vi "HeaderBis.vi"(0 "UUTHeader":string, 1 "ProductRev":string, 2 "P/N UUT":string, 3 "DSP SN":string, 5 "Driver S/N":string, 6 "error in":errorcluster, 10 "UA":string, 11 "VR":string, 12 "POWER SN":string, 13 "Oper.":string, 16 "Revision Param":string, 17 "Tester Software Ver":string) -> (20 "table header":string, 22 "Array":string[][](array[string]), 26 "error out":errorcluster)   [LabVIEW 2017]
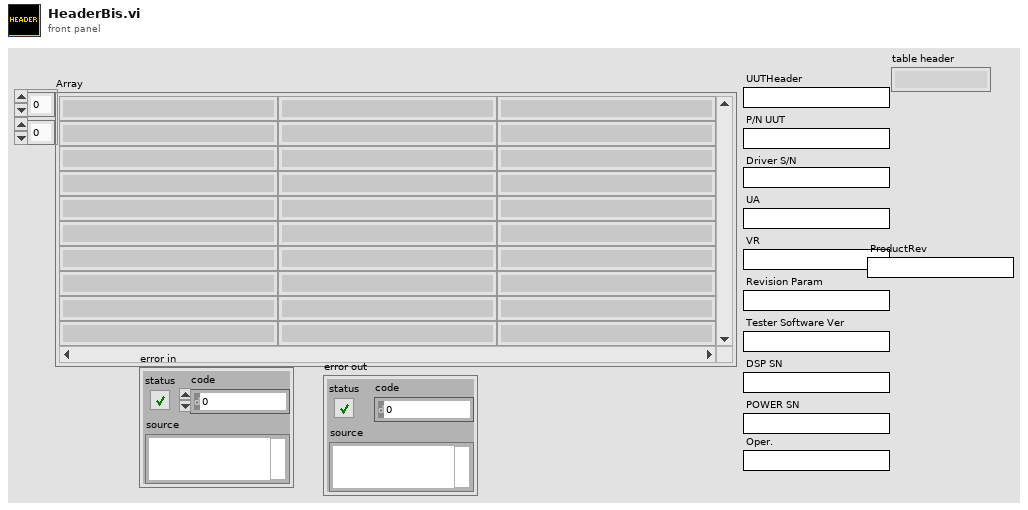
[diagram p1: front panel]
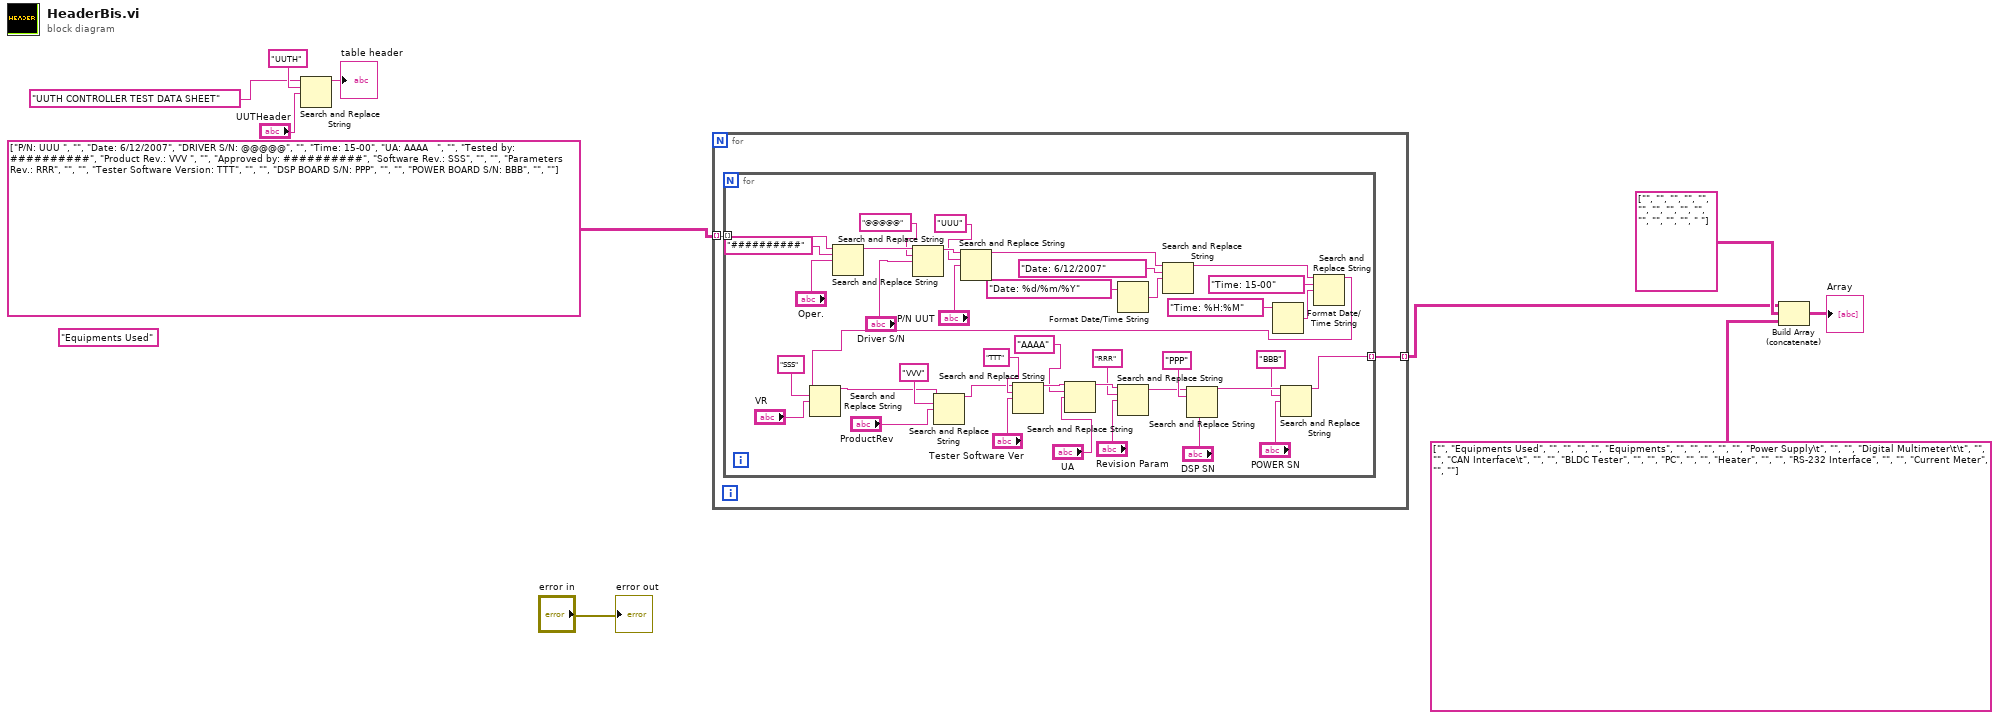
[diagram p0: block diagram]
diagram:
  (unwired) "Equipments Used"
  n1 = Search and Replace String(input string="UUTH CONTROLLER TEST DATA SHEET", search string="UUTH", replace string="UUTHeader") -> (result string=→"table header":string)  [unwired: 5 in, 3 out]
  n2 = for {
    tunnel: string[][] [["P/N: UUU ", "", "Date: 6/12/2007"], ["DRIVER S/N: @@@@@", "", "Time: 15-00"], ["UA: AAAA   ", "", "Tested by: ##########"], ["Product Rev.: VVV ", "", "Approved by: ##########"], ["Software Rev.: SSS", "", ""], ["Parameters Rev.: RRR", "", ""], ["Tester Software Version: TTT", "", ""], ["DSP BOARD S/N: PPP", "", ""], ["POWER BOARD S/N: BBB", "", ""]] -> [w12] mode=indexing
    tunnel: [w11] -> w3 mode=indexing
    n3 = for {
      tunnel: w12 -> [w24] mode=indexing
      tunnel: [w17] -> w11 mode=indexing
      n4 = Search and Replace String(input string=w24, search string="##########" ("source"), replace string="Oper.") -> (result string=w37:string)  [unwired: 5 in, 3 out]
      n5 = Search and Replace String(input string=w37, search string="@@@@@" ("source"), replace string="Driver S/N") -> (result string=w39:string)  [unwired: 5 in, 3 out]
      n6 = Search and Replace String(input string=w39, search string="UUU" ("source"), replace string="P/N UUT") -> (result string=w38:string)  [unwired: 5 in, 3 out]
      n7 = Format Date/Time String(time format string (%c)="Date: %d/%m/%Y") -> (date/time string=w36:string)  [unwired: 2 in]
      n8 = Search and Replace String(input string=w38, search string="Date: 6/12/2007" ("time format string (%c)"), replace string=w36) -> (result string=w47:string)  [unwired: 5 in, 3 out]
      n9 = Format Date/Time String(time format string (%c)="Time: %H:%M") -> (date/time string=w49:string)  [unwired: 2 in]
      n10 = Search and Replace String(input string=w47, search string="Time: 15-00", replace string=w49) -> (result string=w48:string)  [unwired: 5 in, 3 out]
      n11 = Search and Replace String(input string=w48, search string="SSS", replace string="VR") -> (result string=w14:string)  [unwired: 5 in, 3 out]
      n12 = Search and Replace String(input string=w14, search string="VVV", replace string="ProductRev") -> (result string=w13:string)  [unwired: 5 in, 3 out]
      n13 = Search and Replace String(input string=w13, search string="TTT", replace string="Tester Software Ver") -> (result string=w45:string)  [unwired: 5 in, 3 out]
      n14 = Search and Replace String(input string=w45, search string="AAAA", replace string="UA") -> (result string=w51:string)  [unwired: 5 in, 3 out]
      n15 = Search and Replace String(input string=w51, search string="RRR", replace string="Revision Param") -> (result string=w21:string)  [unwired: 5 in, 3 out]
      n16 = Search and Replace String(input string=w21, search string="PPP", replace string="DSP SN") -> (result string=w20:string)  [unwired: 5 in, 3 out]
      n17 = Search and Replace String(input string=w20, search string="BBB", replace string="POWER SN") -> (result string=w17:string)  [unwired: 5 in, 3 out]
    }
  }
  n18 = Build Array (concatenate)(w3, string[][] [["", "", ""], ["", "", ""], ["", "", ""], ["", "", ""], ["", "", " "]], string[][] [["", "Equipments Used", ""], ["", "", ""], ["Equipments", "", ""], ["", "", ""], ["Power Supply\t", "", ""], ["Digital Multimeter\t\t", "", ""], ["CAN Interface\t", "", ""], ["BLDC Tester", "", ""], ["PC", "", ""], ["Heater", "", ""], ["RS-232 Interface", "", ""], ["Current Meter", "", ""]]) -> (→"Array":string[][])
  "error out" <- "error in"
